vi "Set Measurement Name.vi"(0 "Name":string, 11 "error in (no error)":errorcluster) -> (15 "error out":errorcluster)   [LabVIEW 2021, in "Migrator Reusables.lvlib"]
uses:
  Migrator Reusables.lvlib
  controls/Dictionary States.ctl
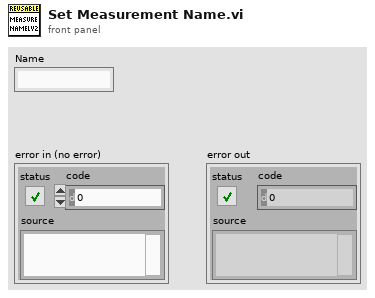
[diagram p1: front panel]
types:
  T1 = typedef "Migrator Reusables.lvlib/Dictionary States.ctl" = enum16{"Set", "Get", "Delete", "Delete All"}
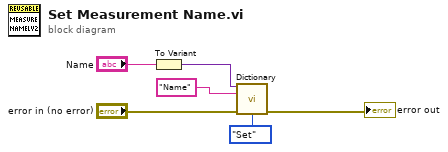
[diagram p0: block diagram]
diagram:
  n1 = To Variant(anything="Name") -> (Variant=w1:variant)
  n2 = call "Dictionary.vi"("Variant_In"=w1, "Key"="Name", "error in (no error)"="error in (no error)", "Dict States"=Dictionary_States."Set") -> ("error out"=→"error out":errorcluster)  [unwired: 10 in, 1 out]
